vi "imagereque.vi"(1 "stop2":bool, 3 "error in":errorcluster, 4 "Time data in":i32[][](array[numeric])) -> (0 "error out":errorcluster, 2 "Time data out":i32[][](array[numeric]), 5 "Frame":i32)   [LabVIEW 2011, in "OfflineTracker.lvlib"]
uses:
  OfflineTracker.lvlib
panel:
  out "Bead":i32
  in  "frame time":i32
  in  "frame number":i32
  in  "state":i32
  in  "bead #":i32
  in  "relative frame #":i32
  in  "xy out":dbl[](array[numeric])
  in  "Image Pixels (U8)":u8[][](array[numeric])
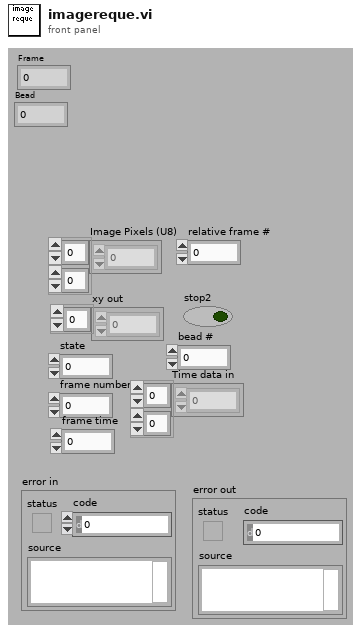
[diagram p1: front panel]
types:
  T1 = typedef "IMAQ Image.ctl" = refnum<image>
  T2 = cluster{"front panel settings":cluster{"files":cluster{"LUT path":path, "Trace path":path, " folders #":i32, "base path":path, "use trace":bool, "use base":bool, "LUT tmp":i32, "Trace tmp":i32, "active path":path}, "Tracking":cluster{"RminZ (pix)":i32, "Rmax (pix)":i32, "angular pixel \ncoverage factor":dbl, "radial pixel \ncoverage factor":dbl}, "Frames":cluster{"Start frame":i32, "number of frames":u32, "display frame ":i32, "track every nd frame ":i32, "Track all frames":bool, "active frame":i32}, "Calibs":cluster{"Zlut number of steps":i32, "pix/um":dbl, "Z correction factor":dbl, "Zlut step size (um)":dbl, "ROI(pix)":i32}, "Beads":cluster{"number of ref beads":i32, "overlay":bool}, "Misc":cluster{"save images to new location":bool, "destination":path}}, "data":cluster{"Image":T1, "image size":i32[], "Bead Array":i32[][], "overlay image":T1, "# beads":i32, "Job list":string[][], "job running":bool, "job #":i32, "folders to go":i32}}
  T3 = cluster{"Image Pixels (U8)":u8[][], "xy out":dbl[], "relative frame #":i32, "bead #":i32, "state":i32, "frame number":i32, "frame time":i32}
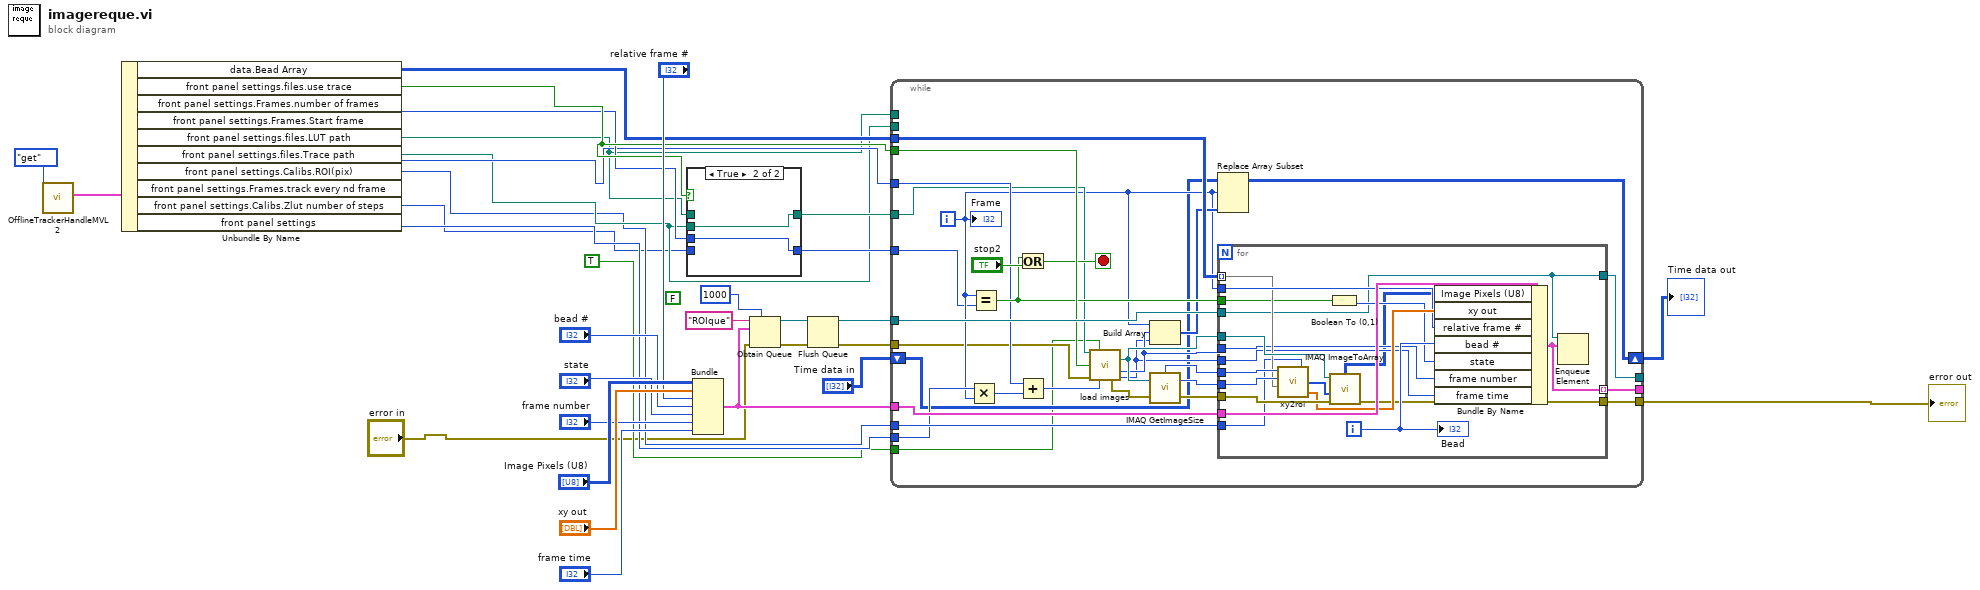
[diagram p0: block diagram]
diagram:
  (unwired) FALSE ("MarijnFormat")
  (unwired) FALSE ("MarijnFormat")
  (unwired) FALSE ("MarijnFormat")
  n1 = call "OfflineTrackerHandleMVL2.vi"("action"=enum16{"get", "set"}."get") -> ("out"=w13:T2)  [unwired: 5 in, 1 out]
  n2 = Unbundle By Name(w13) -> ("data.Bead Array"=w12:i32[][], "front panel settings.files.use trace"=w11:bool, "front panel settings.Frames.number of frames"=w10:u32, "front panel settings.Frames.Start frame"=w9:i32, "front panel settings.files.LUT path"=w8:path, "front panel settings.files.Trace path"=w7:path, "front panel settings.Calibs.ROI(pix)"=w6:i32, "front panel settings.Frames.track every nd frame"=w5:i32, "front panel settings.Calibs.Zlut number of steps"=w4:i32)  [unwired: 1 out]
  n3 = case shown="True" w11 {
    tunnel: w7 -> [_ w36]
    tunnel: [w34 w36] -> w19
    tunnel: w8 -> [w34 _]
    tunnel: w10 -> [_ w35]
    tunnel: w4 -> [w33 _]
    tunnel: [w33 w35] -> w15
    frame False {
    }
    frame True {
    }
  }
  n4 = Bundle("Image Pixels (U8)"="Image Pixels (U8)", "xy out"="xy out", "relative frame #"="relative frame #", "bead #"="bead #", "state"="state", "frame number"="frame number", "frame time"="frame time") -> (w20:T3)  [unwired: 1 out]
  n5 = Obtain Queue(max queue size (-1, unlimited)=1000, name (unnamed)="ROIque", element data type=w20, error in (no error)="error in") -> (queue out=w30:refnum<queue>, error out=w28:errorcluster)  [unwired: 1 in, 1 out]
  n6 = Flush Queue(queue=w30, error in (no error)=w28) -> (queue out=w29:refnum<queue>, error out=w16:errorcluster)  [unwired: 1 out]
  n7 = while {
    tunnel: w29 -> [w61]
    tunnel: w20 -> [w60]
    tunnel: w15 -> [w38]
    tunnel: w9 -> [w52]
    tunnel: w8 -> [_]
    tunnel: w7 -> [_]
    tunnel: w11 -> [w59]
    tunnel: w12 -> [w55]
    tunnel: w6 -> [w54]
    tunnel: w5 -> [w50]
    tunnel: w19 -> [w49]
    shift-right: [w44] -> w17
    shift-left: "Time data in" -> [w43]
    tunnel: [w42] -> _
    tunnel: [w41] -> _
    tunnel: w16 -> [w40]
    tunnel: [w39] -> w1
    tunnel: TRUE ("Use namelist?") -> [w37]
    i -> [w45]
    stop <- w57 stop-if-true
    n8 = Multiply(x=w50, y=w45) -> (x*y=w51:i32)
    n9 = Equal?(x=w45, y=w38) -> (x = y?=w53:bool)
    n10 = Or(x=w53, y="stop2") -> (x .or. y?=w57:bool)
    n11 = Add(x=w52, y=w51) -> (x+y=w58:i32)
    n12 = call "load images.vi"("selected data path"=w49, "DataMarijnFormat"=w37, "Data(T)orLUT(F)?"=w59, "error in"=w40, "frame no."=w58) -> ("Image Out"=w62:T1, "framenumber"=w48:i32, "error out"=w66:errorcluster, "frametime"=w47:i32)  [unwired: 1 in, 6 out]
    n13 = Build Array(w45, w48, w47) -> (w46:i32[])
    n14 = call "IMAQ GetImageSize"("Image"=w62, "error in (no error)"=w66) -> ("Y Resolution"=w63:i32, "X Resolution"=w64:i32, "error out"=w65:errorcluster)  [unwired: 2 out]
    n15 = Replace Array Subset(array=w43, new element=w46, index (row)=w45) -> (w44:i32[][])  [unwired: 1 in]
    n16 = for {
      tunnel: w65 -> [w85]
      tunnel: w64 -> [w84]
      tunnel: w63 -> [w83]
      tunnel: w62 -> [w82]
      tunnel: w61 -> [w70]
      tunnel: w60 -> [w80]
      tunnel: w45 -> [w78]
      tunnel: w55 -> [w77] mode=indexing
      tunnel: w54 -> [w75]
      tunnel: w53 -> [w74]
      tunnel: w48 -> [w72]
      tunnel: w47 -> [w71]
      tunnel: [w70] -> w42
      tunnel: [w69] -> w41 mode=indexing
      tunnel: [w67] -> w39
      i -> [w76]
      n17 = call "xy2roi.vi"("ROI1"=w75, "xy"=w77, "Y Resolution"=w83, "X Resolution"=w84) -> ("xy out"=w79:dbl[], "ROI"=w81:i32[])  [unwired: 1 out]
      n18 = Boolean To (0,1)(Boolean=w74) -> (0, 1=w73:i16)
      n19 = call "IMAQ ImageToArray"("error in (no error)"=w85, "Optional Rectangle"=w81, "Image"=w82) -> ("error out"=w67:errorcluster, "Image Pixels (U8)"=w68:u8[][])  [unwired: 4 out]
      n20 = Bundle By Name(cluster=w80, "Image Pixels (U8)"=w68, "xy out"=w79, "relative frame #"=w78, "bead #"=w76, "state"=w73, "frame number"=w72, "frame time"=w71) -> (w69:T3)
      n21 = Enqueue Element(queue=w70, element=w69) -> ()  [unwired: 1 in, 4 out]
      "Bead" <- w76
    }
    "Frame" <- w45
  }
  "Time data out" <- w17
  "error out" <- w1
